vi "retrieveData.vi"(8 "error in (no error)":errorcluster, 11 "FlukeDMM in":refnum<class "FlukeDMM.lvclass">) -> (0 "error out":errorcluster, 3 "FlukeDMM out":refnum<class "FlukeDMM.lvclass">)   [LabVIEW 2013, in "FlukeDMM.lvlib" / "FlukeDMM.lvclass"]
uses:
  <userlib>/Common/Devices/FlukeDMM/FlukeDMM/FlukeDMM.lvclass
  <userlib>/Common/Devices/FlukeDMM/FlukeDMM/FlukeDMM.lvclass/FlukeDMM.ctl
  <userlib>/Common/SerialProtocols/SerialCommunicator/SerialCommunicator.lvclass
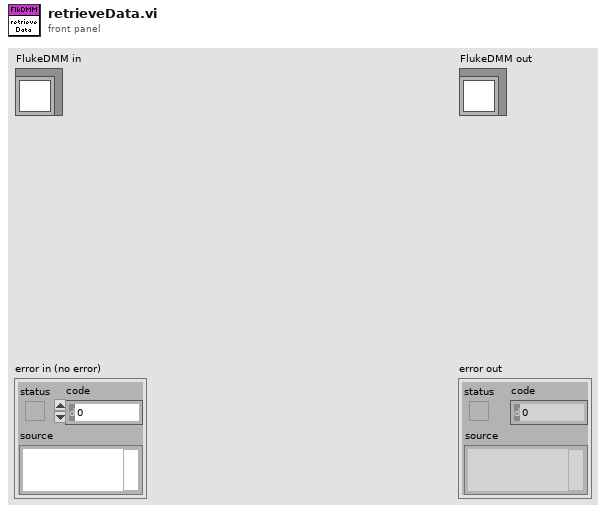
[diagram p1: front panel]
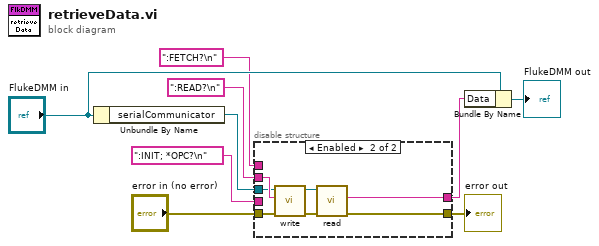
[diagram p0: block diagram]
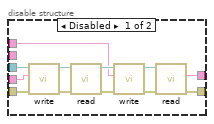
[diagram p2: hidden frame]
diagram:
  n1 = Unbundle By Name("FlukeDMM in") -> ("serialCommunicator"=w9:refnum<class "SerialCommunicator.lvclass">)
  n2 = disable-structure shown="Enabled" {
    disable-tunnel: w9 -> [w21 w25]
    disable-tunnel: "error in (no error)" -> [w20 w24]
    disable-tunnel: [w14 w23] -> w7
    disable-tunnel: ":INIT; *OPC?\n" ("Send") -> [w19 _]
    disable-tunnel: [w10 w22] -> w4
    disable-tunnel: ":FETCH?\n" ("Send") -> [w12 _]
    disable-tunnel: ":READ?\n" ("Send") -> [_ w26]
    frame Disabled {
      n3 = call-dynamic "write.vi"("error in (no error)"=w20, "writeString"=w19, "SerialCommunicator in"=w21) -> ("error out"=w17:errorcluster, "SerialCommunicator out"=w18:refnum<class "SerialCommunicator.lvclass">)  [unwired: 7 in]
      n4 = call-dynamic "read.vi"("error in (no error)"=w17, "SerialCommunicator in"=w18) -> ("error out"=w11:errorcluster, "SerialCommunicator out"=w13:refnum<class "SerialCommunicator.lvclass">)  [unwired: 7 in, 1 out]
      n5 = call-dynamic "write.vi"("error in (no error)"=w11, "writeString"=w12, "SerialCommunicator in"=w13) -> ("error out"=w16:errorcluster, "SerialCommunicator out"=w15:refnum<class "SerialCommunicator.lvclass">)  [unwired: 7 in]
      n6 = call-dynamic "read.vi"("error in (no error)"=w16, "SerialCommunicator in"=w15) -> ("error out"=w14:errorcluster, "stringRead"=w10:string)  [unwired: 7 in, 1 out]
    }
    frame Enabled {
      n7 = call-dynamic "write.vi"("error in (no error)"=w24, "writeString"=w26, "SerialCommunicator in"=w25) -> ("error out"=w27:errorcluster, "SerialCommunicator out"=w28:refnum<class "SerialCommunicator.lvclass">)  [unwired: 7 in]
      n8 = call-dynamic "read.vi"("error in (no error)"=w27, "SerialCommunicator in"=w28) -> ("error out"=w23:errorcluster, "stringRead"=w22:string)  [unwired: 7 in, 1 out]
    }
  }
  "error out" <- w7
  n9 = Bundle By Name(cluster="FlukeDMM in", "Data"=w4) -> (→"FlukeDMM out":refnum<class "FlukeDMM.lvclass">)
